vi "Is Type.vi"(10 "Type":refnum<class>, 11 "Value":refnum<class>) -> (2 "Type Matches":bool, 3 "Value Class":string)   [LabVIEW 2023, in "Promises.lvlib"]
uses:
  Promises.lvlib
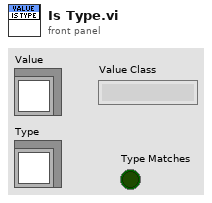
[diagram p1: front panel]
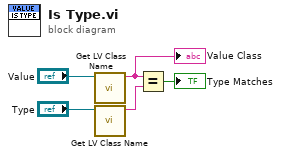
[diagram p0: block diagram]
diagram:
  n1 = call <vilib>:"Get LV Class Name.vi"("object"="Value") -> ("class name"=w1:string)  [unwired: 9 in, 1 out]
  "Value Class" <- w1
  n2 = call <vilib>:"Get LV Class Name.vi"("object"="Type") -> ("class name"=w5:string)  [unwired: 9 in, 1 out]
  n3 = Equal?(x=w1, y=w5) -> (x = y?=→"Type Matches":bool)
